vi "Code Benchmark Template.vi"() -> ()   [LabVIEW 2017]
doc: "Use this template to build a VI to use as a subVI."
uses:
  <userlib>/_OpenG.lib/md5/md5.llb/MD5 Message Digest (Binary String)__ogtk.vi
panel:
  out "unit (ms)":dbl[](graph)
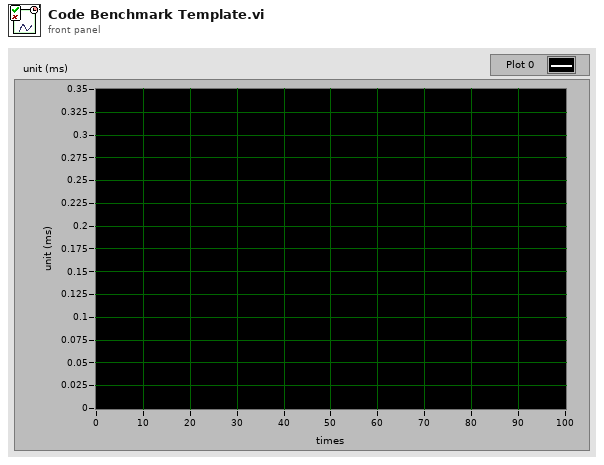
[diagram p1: front panel]
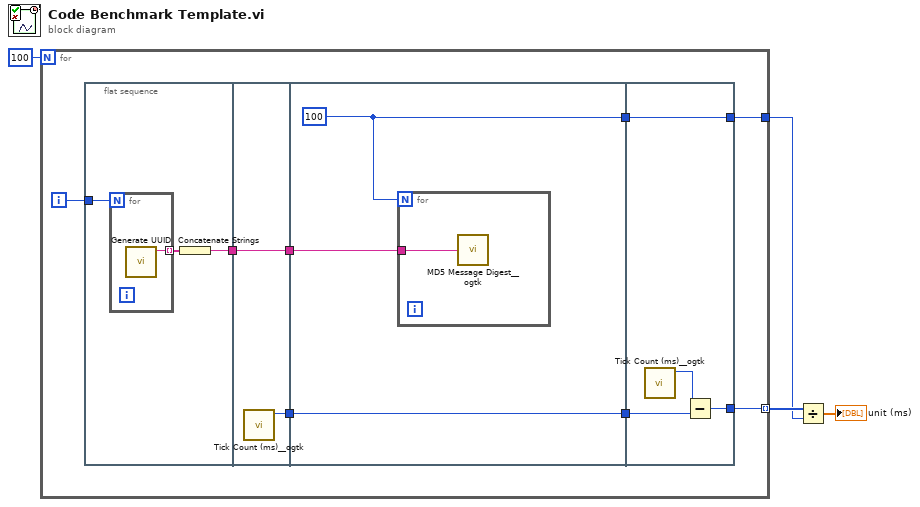
[diagram p0: block diagram]
diagram:
  n1 = for {
    N: 100 -> [_]
    tunnel: [w10] -> w2 mode=indexing
    tunnel: [w9] -> w1
    i -> [w7]
    n2 = flat-sequence {
      tunnel: w7 -> [w15]
      tunnel: [w13] -> w5
      tunnel: [w18] -> w12
      tunnel: [w17] -> w6
      tunnel: w5 -> [w17]
      tunnel: w12 -> [w21]
      tunnel: [w21] -> w11
      tunnel: [w20] -> w8
      tunnel: w6 -> [w19]
      tunnel: w11 -> [w25]
      tunnel: [w24] -> w10
      tunnel: [w23] -> w9
      tunnel: w8 -> [w23]
      frame #0 {
        n3 = for {
          N: w15 -> [_]
          tunnel: [w16] -> w14 mode=indexing
          n4 = call "Generate UUID.vi"() -> ("UUID"=w16:string)  [unwired: 11 in]
        }
        n5 = Concatenate Strings(w14) -> (w13:string)
      }
      frame #1 {
        n6 = call <userlib>:"Tick Count (ms)__ogtk.vi"() -> ("millisecond timer value"=w18:u32)  [unwired: 10 in, 1 out]
      }
      frame #2 {
        w20 = 100
        n7 = for {
          N: w20 -> [_]
          tunnel: w19 -> [w22]
          n8 = call-poly <userlib>:"MD5 Message Digest__ogtk.vi"("Message"=w22) -> ()  [unwired: 1 out]
        }
      }
      frame #3 {
        n9 = call <userlib>:"Tick Count (ms)__ogtk.vi"() -> ("millisecond timer value"=w26:u32)  [unwired: 10 in, 1 out]
        n10 = Subtract(x=w26, y=w25) -> (x-y=w24:u32)
      }
    }
  }
  n11 = Divide(x=w2, y=w1) -> (x/y=→"unit (ms)":dbl[])
